vi "Polar to Arrow.vi"(8 "error in":errorcluster, 9 "Phases [rad]":dbl[](array[numeric]), 10 "Magnitudes":dbl[](array[numeric])) -> (0 "error out":errorcluster, 1 "Vector coordinates":cluster{"Real":dbl[], "Imag":dbl[]}[](array[cluster]), 2 "z":cdb[](array[numeric]))   [LabVIEW 2020]
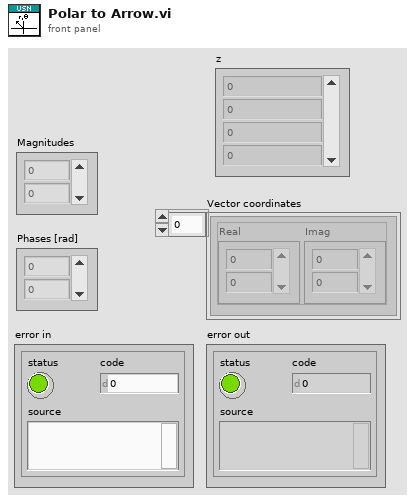
[diagram p1: front panel]
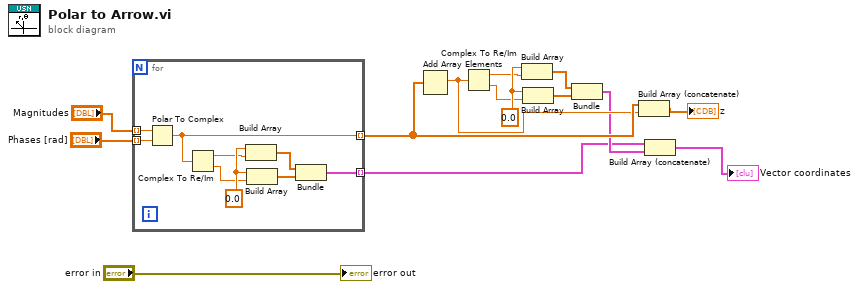
[diagram p0: block diagram]
diagram:
  w11 = 0.0
  n1 = for {
    tunnel: "Magnitudes" -> [w18] mode=indexing
    tunnel: "Phases [rad]" -> [w17] mode=indexing
    tunnel: [w16] -> w2 mode=indexing
    tunnel: [w15] -> w6 mode=indexing
    w23 = 0.0
    n2 = Polar To Complex(1:w17, 2:w18) -> (0:w15:cdb)
    n3 = Complex To Re/Im(x + iy=w15) -> (x=w21:dbl, y=w22:dbl)
    n4 = Build Array(w23, w21) -> (w19:dbl[])
    n5 = Build Array(w23, w22) -> (w20:dbl[])
    n6 = Bundle(w19, w20) -> (w16:cluster{dbl[], dbl[]})  [unwired: 1 in]
  }
  n7 = Add Array Elements(numeric array=w6) -> (sum=w5:cdb)
  n8 = Complex To Re/Im(x + iy=w5) -> (x=w9:dbl, y=w10:dbl)
  n9 = Build Array(w11, w9) -> (w7:dbl[])
  n10 = Build Array(w11, w10) -> (w8:dbl[])
  n11 = Bundle(w7, w8) -> (w3:cluster{dbl[], dbl[]})  [unwired: 1 in]
  n12 = Build Array (concatenate)(w6, w5) -> (→"z":cdb[])
  n13 = Build Array (concatenate)(w2, w3) -> (→"Vector coordinates":cluster{dbl[], dbl[]}[])
  "error out" <- "error in"
